vi "TON.vi"(9 "Delay (ms)":u32=500, 10 "Input":bool) -> (2 "Output":bool)   [LabVIEW 2015]
doc: "The TON, when given a True input, will wait for the specified delay to elapse before outputting True. When the input reverts back to False, the output will immediately revert back to false."
panel:
  in  "Delay_TON":T1
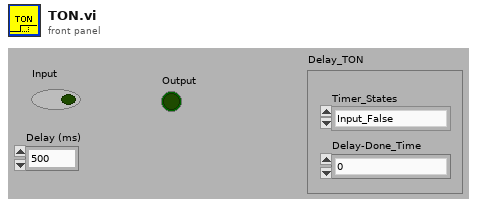
[diagram p1: front panel]
types:
  T1 = cluster{"Timer_States":enum16{"Input_False", "Input_True_Start_Timing", "Input_True_Timing", "Input_True_Timing_Complete"}, "Delay-Done_Time":u32}
  T2 = enum16{"Input_False", "Input_True_Start_Timing", "Input_True_Timing", "Input_True_Timing_Complete"}
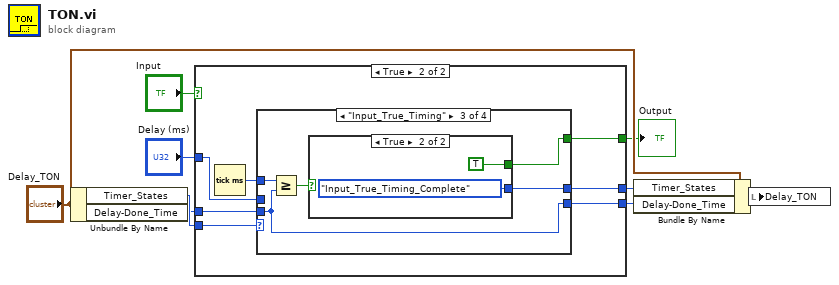
[diagram p0: block diagram]
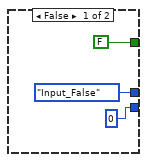
[diagram p2: hidden frame]
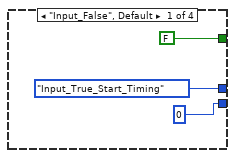
[diagram p3: hidden frame]
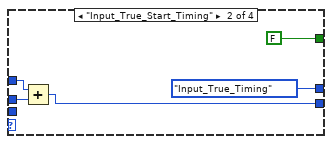
[diagram p4: hidden frame]
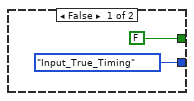
[diagram p5: hidden frame]
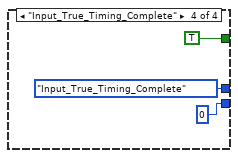
[diagram p6: hidden frame]
diagram:
  n1 = Unbundle By Name("Delay_TON") -> ("Timer_States"=w8:T2, "Delay-Done_Time"=w4:u32)
  n2 = case shown="True" "Input" {
    tunnel: [FALSE ("Boolean 2") w14] -> w1
    tunnel: w8 -> [_ w13]
    tunnel: [T2."Input_False" ("Timer_States") w19] -> w7
    tunnel: [u32 0 ("Delay-Done_Time") w18] -> w6
    tunnel: "Delay (ms)" -> [_ w16]
    tunnel: w4 -> [_ w15]
    frame False {
    }
    frame True {
      n3 = Tick Count (ms)() -> (millisecond timer value=w17:u32)
      n4 = case shown="\"Input_True_Timing\"" w13 {
        tunnel: [T2."Input_True_Start_Timing" ("Timer_States") T2."Input_True_Timing" ("Timer_States") w30 T2."Input_True_Timing_Complete" ("Timer_States")] -> w19
        tunnel: [u32 0 ("Delay-Done_Time") w25 w28 u32 0 ("Delay-Done_Time")] -> w18
        tunnel: w17 -> [_ w27 w32 _]
        tunnel: w16 -> [_ w26 _ _]
        tunnel: w15 -> [_ _ w28 _]
        tunnel: [FALSE ("DOUT-TON") FALSE ("DOUT-TON") w29 TRUE ("DOUT-TON")] -> w14
        frame "Input_False", Default {
        }
        frame "Input_True_Start_Timing" {
          n5 = Add(x=w27, y=w26) -> (x+y=w25:u32)
        }
        frame "Input_True_Timing" {
          n6 = Greater Or Equal?(x=w32, y=w28) -> (x >= y?=w31:bool)
          n7 = case shown="True" w31 {
            tunnel: [T2."Input_True_Timing" ("Timer_States") T2."Input_True_Timing_Complete" ("Timer_States")] -> w30
            tunnel: [FALSE TRUE] -> w29
            frame False {
            }
            frame True {
            }
          }
        }
        frame "Input_True_Timing_Complete" {
        }
      }
    }
  }
  "Output" <- w1
  n8 = Bundle By Name(cluster="Delay_TON", "Timer_States"=w7, "Delay-Done_Time"=w6) -> (w2:T1)
  n9 = local write "Delay_TON"(w2) -> ()
